vi "TakeThirdTote.vi"(11 "Array":bool[](array[boolean])) -> ()   [LabVIEW 2014]
uses:
  TakeThirdTote.ctl
  Gantry/GantryGlobals.vi
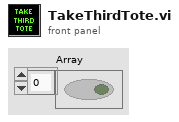
[diagram p1: front panel]
types:
  T1 = typedef "TakeThirdTote.ctl" = enum16{"WaitingForInput", "RaiseLift", "GantryOut", "CloseArms", "LiftUpALittle", "GantryIn", "LowerLift"}
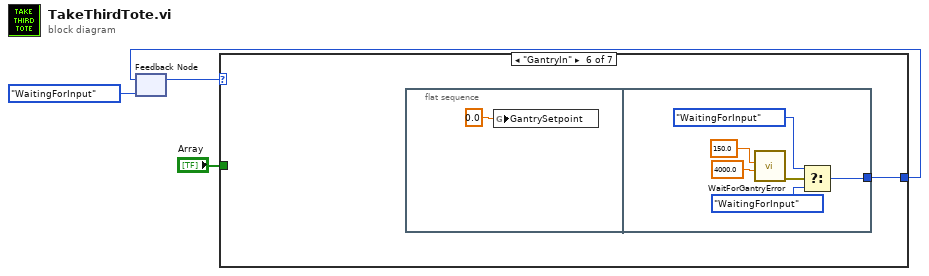
[diagram p0: block diagram]
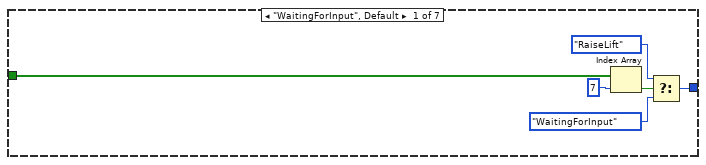
[diagram p2: hidden frame]
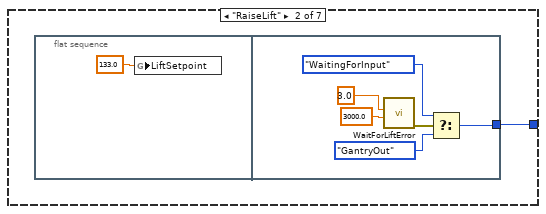
[diagram p3: hidden frame]
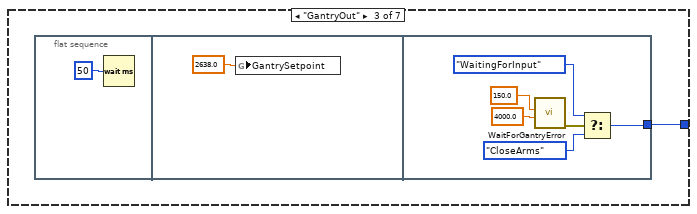
[diagram p4: hidden frame]
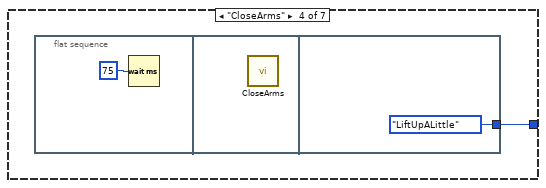
[diagram p5: hidden frame]
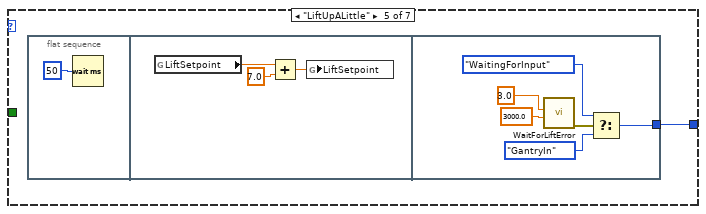
[diagram p6: hidden frame]
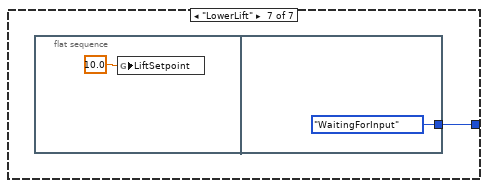
[diagram p7: hidden frame]
diagram:
  n1 = feedback #1(TakeThirdTote."WaitingForInput" ("Enum")) -> (w4:T1)
  n2 = case shown="\"GantryIn\"" w4 {
    tunnel: "Array" -> [w6 _ _ _ _ _ _]
    tunnel: [w5 w11 w19 w28 w31 w42 w50] -> w1
    frame "WaitingForInput", Default {
      n3 = Index Array(array=w6, index=7) -> (element=w9:bool)
      n4 = Select(t=TakeThirdTote."RaiseLift" ("Enum"), s=w9, f=TakeThirdTote."WaitingForInput" ("Enum")) -> (s? t:f=w5:T1)
    }
    frame "RaiseLift" {
      n5 = flat-sequence {
        tunnel: [w13] -> w11
        frame #0 {
          n6 = global write "GantryGlobals.vi" "LiftSetpoint"(133.0 ("LiftSetpoint")) -> ()
        }
        frame #1 {
          n7 = call "WaitForLiftError.vi"("Timeout (ms)"=3000.0, "AllowedError"=3.0) -> ("error out"=w16:errorcluster)  [unwired: 9 in]
          n8 = Select(t=TakeThirdTote."WaitingForInput" ("Enum"), s=w16, f=TakeThirdTote."GantryOut" ("Enum")) -> (s? t:f=w13:T1)
        }
      }
    }
    frame "GantryOut" {
      n9 = flat-sequence {
        tunnel: [w22] -> w19
        frame #0 {
          n10 = Wait (ms)(milliseconds to wait=u32 50) -> ()  [unwired: 1 out]
        }
        frame #1 {
          n11 = global write "GantryGlobals.vi" "GantrySetpoint"(2638.0 ("GantrySetpoint")) -> ()
        }
        frame #2 {
          n12 = call "WaitForGantryError.vi"("Timeout (ms)"=4000.0, "AllowedError"=150.0) -> ("error out"=w25:errorcluster)  [unwired: 9 in]
          n13 = Select(t=TakeThirdTote."WaitingForInput" ("Enum"), s=w25, f=TakeThirdTote."CloseArms" ("Enum")) -> (s? t:f=w22:T1)
        }
      }
    }
    frame "CloseArms" {
      n14 = flat-sequence {
        tunnel: [TakeThirdTote."LiftUpALittle" ("Enum")] -> w28
        frame #0 {
          n15 = Wait (ms)(milliseconds to wait=u32 75) -> ()  [unwired: 1 out]
        }
        frame #1 {
          n16 = call "CloseArms.vi"() -> ()  [unwired: 12 in]
        }
        frame #2 {
        }
      }
    }
    frame "LiftUpALittle" {
      n17 = flat-sequence {
        tunnel: [w36] -> w31
        frame #0 {
          n18 = Wait (ms)(milliseconds to wait=u32 50) -> ()  [unwired: 1 out]
        }
        frame #1 {
          n19 = global read "GantryGlobals.vi" "LiftSetpoint"() -> (w35:dbl)
          n20 = Add(x=w35, y=7.0) -> (x+y=w33:dbl)
          n21 = global write "GantryGlobals.vi" "LiftSetpoint"(w33) -> ()
        }
        frame #2 {
          n22 = call "WaitForLiftError.vi"("Timeout (ms)"=3000.0, "AllowedError"=3.0) -> ("error out"=w39:errorcluster)  [unwired: 9 in]
          n23 = Select(t=TakeThirdTote."WaitingForInput" ("Enum"), s=w39, f=TakeThirdTote."GantryIn" ("Enum")) -> (s? t:f=w36:T1)
        }
      }
    }
    frame "GantryIn" {
      n24 = flat-sequence {
        tunnel: [w44] -> w42
        frame #0 {
          n25 = global write "GantryGlobals.vi" "GantrySetpoint"(0.0 ("GantrySetpoint")) -> ()
        }
        frame #1 {
          n26 = call "WaitForGantryError.vi"("Timeout (ms)"=4000.0, "AllowedError"=150.0) -> ("error out"=w47:errorcluster)  [unwired: 9 in]
          n27 = Select(t=TakeThirdTote."WaitingForInput" ("Enum"), s=w47, f=TakeThirdTote."WaitingForInput" ("Enum")) -> (s? t:f=w44:T1)
        }
      }
    }
    frame "LowerLift" {
      n28 = flat-sequence {
        tunnel: [TakeThirdTote."WaitingForInput" ("Enum")] -> w50
        frame #0 {
          n29 = global write "GantryGlobals.vi" "LiftSetpoint"(10.0 ("LiftSetpoint")) -> ()
        }
        frame #1 {
        }
      }
    }
  }
  n30 = feedback-in #1(w1) -> ()
